vi "FFTinv r,Theta to x(t)_Ch3.vi"(8 "Nyquist Freq. Phase (Radians)":dbl format="%.2f", 9 "Nyquist Freq. Mag (Linear)":dbl format="%.2f", 10 "+Freq Phase of FFT (Radians)":dbl[](array[numeric]) format="%.2f", 11 "+Freq. Mag of FFT (Linear)":dbl[](array[numeric]) format="%.2f") -> (3 "X(t)":dbl[](array[numeric]) format="%.2f", 4 "error":i32)   [LabVIEW 2015]
uses:
  <vilib>/Analysis/NI_AALPro.lvlib
  <vilib>/Analysis/2dsp.llb/Inverse Real FFT.vi
panel:
  out "input Data Error":bool
  out "Numeric 2":dbl
  out "Numeric":dbl
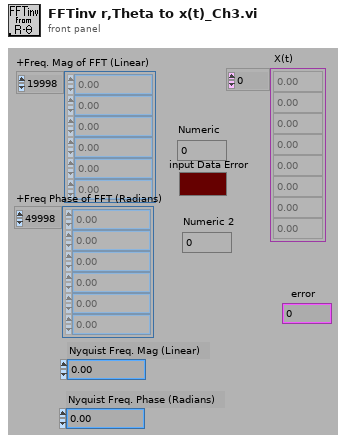
[diagram p1: front panel]
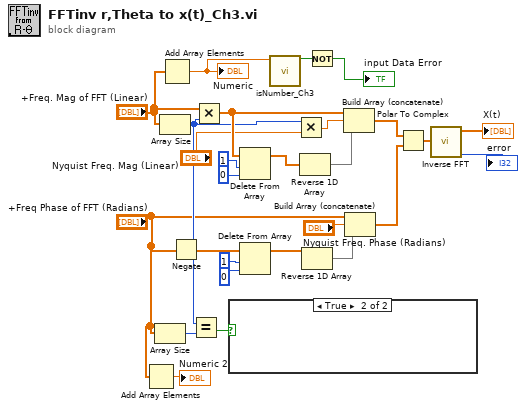
[diagram p0: block diagram]
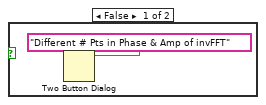
[diagram p2: hidden frame]
diagram:
  n1 = Add Array Elements(numeric array="+Freq Phase of FFT (Radians)") -> (sum=→"Numeric 2":dbl)
  n2 = Array Size(array="+Freq Phase of FFT (Radians)") -> (size(s)=w7:i32)
  n3 = Array Size(array="+Freq. Mag of FFT (Linear)") -> (size(s)=w8:i32)
  n4 = Add Array Elements(numeric array="+Freq. Mag of FFT (Linear)") -> (sum=w3:dbl)
  "Numeric" <- w3
  n5 = Negate(x="+Freq Phase of FFT (Radians)") -> (-x=w24:dbl[])
  n6 = Equal?(x=w8, y=w7) -> (x = y?=w9:bool)
  n7 = Multiply(x="+Freq. Mag of FFT (Linear)", y=w8) -> (x*y=w27:dbl[])
  n8 = case shown="True" w9 {
    frame False {
      n9 = Two Button Dialog(message="Different # Pts in Phase & Amp of invFFT") -> ()  [unwired: 2 in, 1 out]
    }
    frame True {
    }
  }
  n10 = Delete From Array(array=w27, length=1, index=0) -> (array with subset deleted=w26:dbl[])  [unwired: 1 out]
  n11 = Delete From Array(array=w24, length=1, index=0) -> (array with subset deleted=w20:dbl[])  [unwired: 1 out]
  n12 = call "isNumber_Ch3.vi"("\"Number\" in question"=w3) -> ("n=is a number"=w2:bool)  [unwired: 8 in, 2 out]
  n13 = Multiply(x=w8, y="Nyquist Freq. Mag (Linear)") -> (x*y=w11:dbl)
  n14 = Reverse 1D Array(array=w26) -> (reversed array=w25:dbl[])
  n15 = Reverse 1D Array(array=w20) -> (reversed array=w21:dbl[])
  n16 = Not(x=w2) -> (.not. x?=→"input Data Error":bool)
  n17 = Build Array (concatenate)(w27, w11, w25) -> (w23:dbl[])
  n18 = Build Array (concatenate)("+Freq Phase of FFT (Radians)", "Nyquist Freq. Phase (Radians)", w21) -> (w22:dbl[])
  n19 = Polar To Complex(1:w22, 2:w23) -> (0:w14:cdb[])
  n20 = call-poly <vilib>:"Inverse FFT.vi"("FFT {X}"=w14) -> ("error"=→"error":i32, "X"=→"X(t)":dbl[])  [unwired: 9 in]
